vi "Write Comparison Type.vi"(8 "error in (no error)":errorcluster, 10 "Comparison Type":string, 11 "Result in":refnum<class "Result.lvclass">) -> (0 "error out":errorcluster, 3 "Result out":refnum<class "Result.lvclass">)   [LabVIEW 2015, in "Result.lvclass"]
uses:
  Result.lvclass
  Result.lvclass/Result.ctl
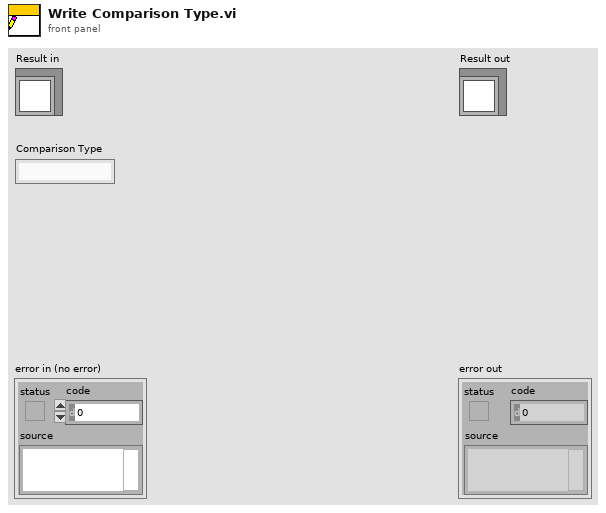
[diagram p1: front panel]
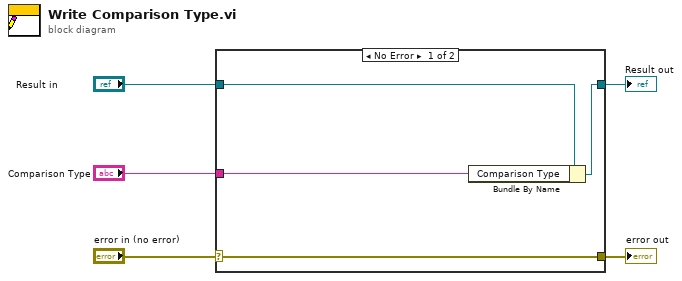
[diagram p0: block diagram]
diagram:
  n1 = case shown="No Error" "error in (no error)" {
    selector: "error in (no error)" -> [w9 w10]
    tunnel: [w9 w10] -> w4
    tunnel: [w7 w11] -> w2
    tunnel: "Result in" -> [w8 w11]
    tunnel: "Comparison Type" -> [w6 _]
    frame No Error {
      n2 = Bundle By Name(cluster=w8, "Comparison Type"=w6) -> (w7:refnum<class "Result.lvclass">)
    }
    frame Error {
    }
  }
  "error out" <- w4
  "Result out" <- w2
